vi "get_specified_representation.vi"(11 "Control Data Type":T1) -> (2 "Format String":string, 3 "Representation":T2(ring))   [LabVIEW 2018]
uses:
  TypeDefinitions/control_data_type.ctl
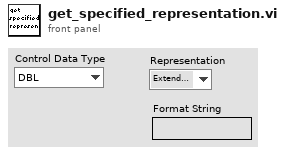
[diagram p1: front panel]
types:
  T1 = typedef "control_data_type.ctl" = enum16{"DBL", "I32", "Boolean", "String", "U16", "U32", "EXT", "SGL", "I16", "U8", "I8", "I64", "U64", "Waveform", "Reference", "Variant", "Cluster"}
  T2 = enum32{"Extended Precision", "Double Precision", "Single Precision", "Long", "Word", "Byte", "Unsigned Long", "Unsigned Word", "Unsigned Byte", "Complex Extended", "Complex Double", "Complex Single", "Quad", "Unsigned Quad", "Fixed-Point"}
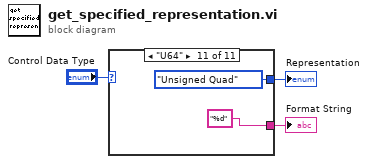
[diagram p0: block diagram]
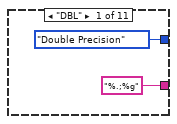
[diagram p2: hidden frame]
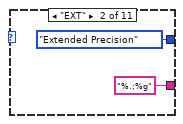
[diagram p3: hidden frame]
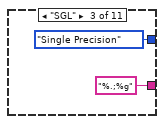
[diagram p4: hidden frame]
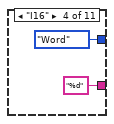
[diagram p5: hidden frame]
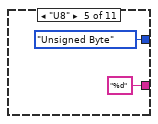
[diagram p6: hidden frame]
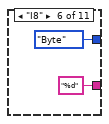
[diagram p7: hidden frame]
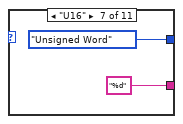
[diagram p8: hidden frame]
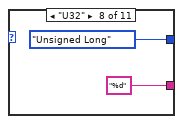
[diagram p9: hidden frame]
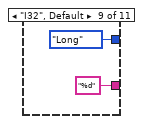
[diagram p10: hidden frame]
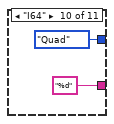
[diagram p11: hidden frame]
diagram:
  n1 = case shown="\"U64\"" "Control Data Type" {
    tunnel: [T2."Double Precision" ("Representation") T2."Extended Precision" ("Representation") T2."Single Precision" ("Representation") T2."Word" ("Representation") T2."Unsigned Byte" ("Representation") T2."Byte" ("Representation") T2."Unsigned Word" ("Representation") T2."Unsigned Long" ("Representation") T2."Long" ("Representation") T2."Quad" ("Representation") T2."Unsigned Quad" ("Representation")] -> w3
    tunnel: ["%.;%g" "%.;%g" "%.;%g" "%d" "%d" "%d" "%d" "%d" "%d" "%d" "%d"] -> w1
    frame "DBL" {
    }
    frame "EXT" {
    }
    frame "SGL" {
    }
    frame "I16" {
    }
    frame "U8" {
    }
    frame "I8" {
    }
    frame "U16" {
    }
    frame "U32" {
    }
    frame "I32", Default {
    }
    frame "I64" {
    }
    frame "U64" {
    }
  }
  "Representation" <- w3
  "Format String" <- w1
